vi "GetLatestDataPack.vi"(8 "error in (no error)":errorcluster, 11 "reference in":refnum<k24>) -> (0 "error out":errorcluster, 2 "LatestDataPackage":refnum<k24>, 3 "reference out":refnum<k24>)   [LabVIEW 2019, in "LabNation Scope Driver.lvlib"]
doc: "Acquires a handle to the latest acquired data package from the scope."
uses:
  LabNation Scope Driver.lvlib
  C:/Program Files (x86)/LabNation/SmartScope/DeviceInterface.dll
  Program Files (x86)/LabNation/SmartScope/DeviceInterface.dll
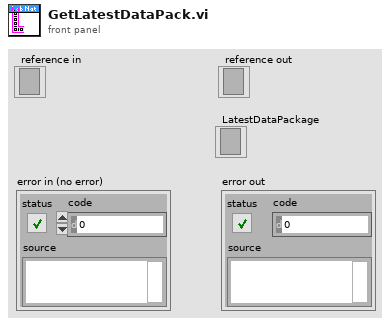
[diagram p1: front panel]
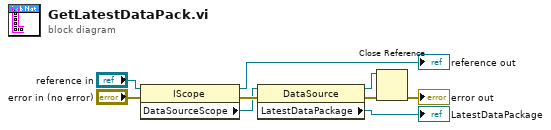
[diagram p0: block diagram]
diagram:
  n1 = property class="IScope"(reference="reference in", error in="error in (no error)") -> (reference out=→"reference out":refnum<k24>, error out=w8:errorcluster, "DataSourceScope"=w4:refnum<k24>)
  n2 = property class="DataSource"(reference=w4, error in=w8) -> (reference out=w1:refnum<k24>, error out=w7:errorcluster, "LatestDataPackage"=→"LatestDataPackage":refnum<k24>)
  n3 = Close Reference(reference=w1, error in (no error)=w7) -> (error out=→"error out":errorcluster)
